vi "Perform_Analysis.vi"(5 "Std Dev in":dbl=0.04 format="%0.2f", 6 "Std Dev 3":dbl=0.005 format="%0.2f", 7 "Array 2":dbl[](array[numeric]), 8 "Common std dev":dbl=0.4 format="%0.2f", 9 "Array":dbl[](array[numeric]), 10 "Nb of samples":i32=10000 min=0 max=50000, 11 "IntensityGraph in":refnum<vi>) -> (1 "Histogram":u32[](graph), 2 "Intensity Graph":u32[][](graph), 3 "Scatter Plot":cluster{dbl[], dbl[]}(graph))   [LabVIEW 2015]
uses:
  ESA_Data_Analysis_Global_VIs.vi
  <vilib>/ptbypt/NI_PtbyPt.lvlib
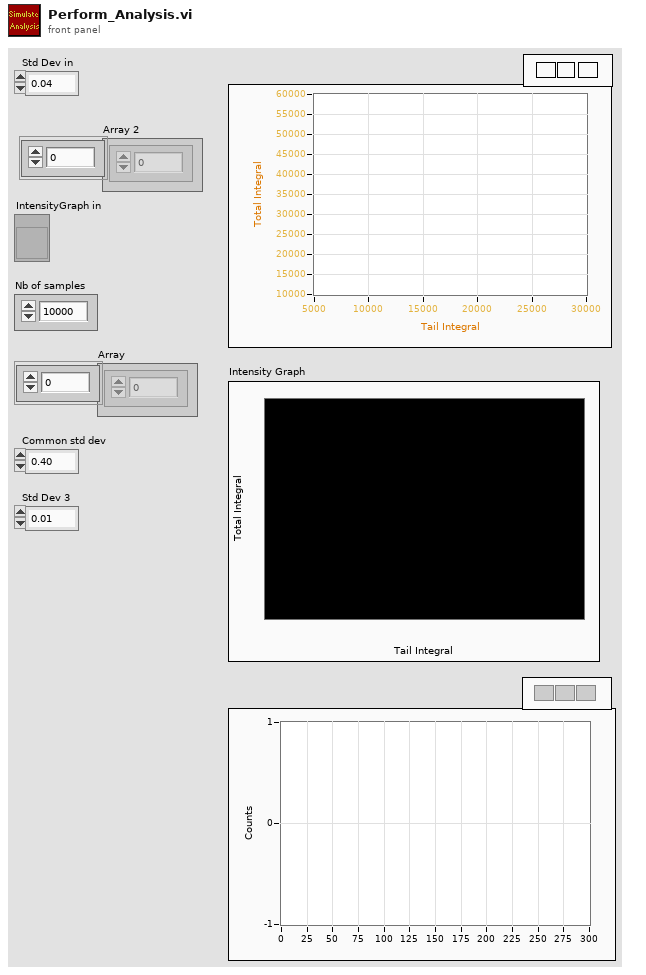
[diagram p1: front panel]
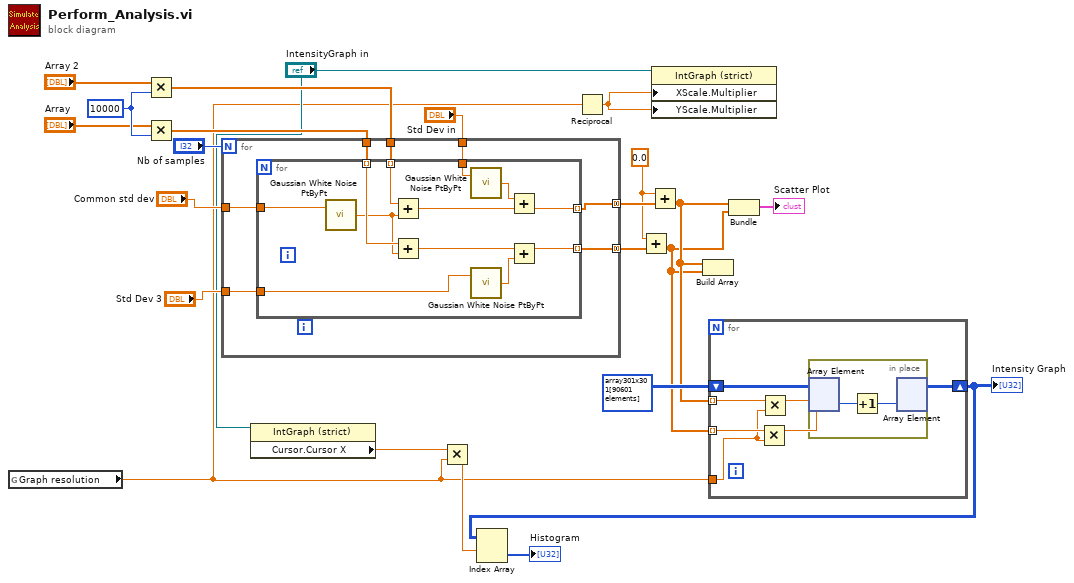
[diagram p0: block diagram]
diagram:
  w2 = 0.0
  w8 = 10000
  n1 = global read "ESA_Data_Analysis_Global_VIs.vi" "Graph resolution"() -> (w1:dbl)
  n2 = Multiply(x="Array 2", y=w8) -> (x*y=w9:dbl[])
  n3 = Multiply(x="Array", y=w8) -> (x*y=w10:dbl[])
  n4 = for {
    N: "Nb of samples" -> [_]
    tunnel: w9 -> [w30]
    tunnel: w10 -> [w29]
    tunnel: [w28] -> w14 mode=concatenating
    tunnel: [w27] -> w15 mode=concatenating
    tunnel: "Common std dev" -> [w26]
    tunnel: "Std Dev 3" -> [w25]
    tunnel: "Std Dev in" -> [w24]
    n5 = for {
      tunnel: w30 -> [w42] mode=indexing
      tunnel: w29 -> [w41] mode=indexing
      tunnel: [w38] -> w28 mode=indexing
      tunnel: [w36] -> w27 mode=indexing
      tunnel: w26 -> [w33]
      tunnel: w25 -> [w32]
      tunnel: w24 -> [w31]
      n6 = call <vilib>:"Gaussian White Noise PtByPt.vi"("standard deviation"=w33) -> ("Gaussian white noise"=w34:dbl)  [unwired: 2 in]
      n7 = Add(x=w42, y=w34) -> (x+y=w40:dbl)
      n8 = Add(x=w41, y=w34) -> (x+y=w39:dbl)
      n9 = call <vilib>:"Gaussian White Noise PtByPt.vi"("standard deviation"=w31) -> ("Gaussian white noise"=w37:dbl)  [unwired: 2 in]
      n10 = call <vilib>:"Gaussian White Noise PtByPt.vi"("standard deviation"=w32) -> ("Gaussian white noise"=w35:dbl)  [unwired: 2 in]
      n11 = Add(x=w37, y=w40) -> (x+y=w38:dbl)
      n12 = Add(x=w39, y=w35) -> (x+y=w36:dbl)
    }
  }
  n13 = property on="Property Node" class="IntGraph (strict)"(reference="IntensityGraph in") -> ("Cursor.Cursor X"=w19:dbl)  [unwired: 1 in, 2 out]
  n14 = Multiply(x=w19, y=w1) -> (x*y=w20:dbl)
  n15 = Reciprocal(x=w1) -> (1/x=w13:dbl)
  n16 = Add(x=w2, y=w15) -> (x+y=w3:dbl[])
  n17 = Add(x=w2, y=w14) -> (x+y=w4:dbl[])
  n18 = property on="Property Node" class="IntGraph (strict)"(reference="IntensityGraph in", "XScale.Multiplier"=w13, "YScale.Multiplier"=w13) -> ()  [unwired: 1 in, 2 out]
  n19 = Build Array(w4, w3) -> ()  [unwired: 1 out]
  n20 = for {
    shift-right: [w48] -> w17
    shift-left: u32[][] array301x301[90601 elements] -> [w49]
    tunnel: w4 -> [w47] mode=indexing
    tunnel: w3 -> [w46] mode=indexing
    tunnel: w1 -> [w43]
    n21 = Multiply(x=w46, y=w43) -> (x*y=w44:dbl)
    n22 = Multiply(x=w47, y=w43) -> (x*y=w45:dbl)
    n23 = in-place {
      n24 = in-place-array #1(w49, w45, w44) -> (w51:u32)
      n25 = Increment(x=w51) -> (x+1=w50:u32)
      n26 = in-place-array #1(w50) -> (w48:u32[][])  [unwired: 2 out]
    }
  }
  "Intensity Graph" <- w17
  n27 = Index Array(array=w17, index (row)=w20) -> (element=→"Histogram":u32[])  [unwired: 1 in]
  n28 = Bundle(w4, w3) -> (→"Scatter Plot":cluster{dbl[], dbl[]})  [unwired: 1 in]
